vi "GenCM-Read connections.vi"(0 "AO Map":T1, 1 "Path":path, 5 "AI Map":T1, 7 "Digital I-O ref":refnum<vi>, 9 "slot ctl refs":refnum<vi>[](array[refnum]), 11 "error in (no error)":errorcluster, 12 "Analog":cluster{"Inputs":string[], "Outputs":string[]}, 13 "Digital":cluster{"Inputs":string[], "Outputs":string[]}) -> (4 "Hide unused?":bool, 10 "slot ctl refs out":refnum<vi>[](array[refnum]), 15 "error out":errorcluster)   [LabVIEW 2015]
uses:
  Type Defs/General PXISlot XControl/PXISlotGP.xctl
  Type Defs/Digital I-O XControl/Digital I-O.xctl
  PXI DAQ VIs/Utility VIs/Array Dimensions (2D).vi
  <vilib>/Utility/config.llb/Read Key (I32).vi
  <vilib>/Utility/config.llb/Read Key (Boolean).vi
  <vilib>/Utility/config.llb/NI_LVConfig.lvlib
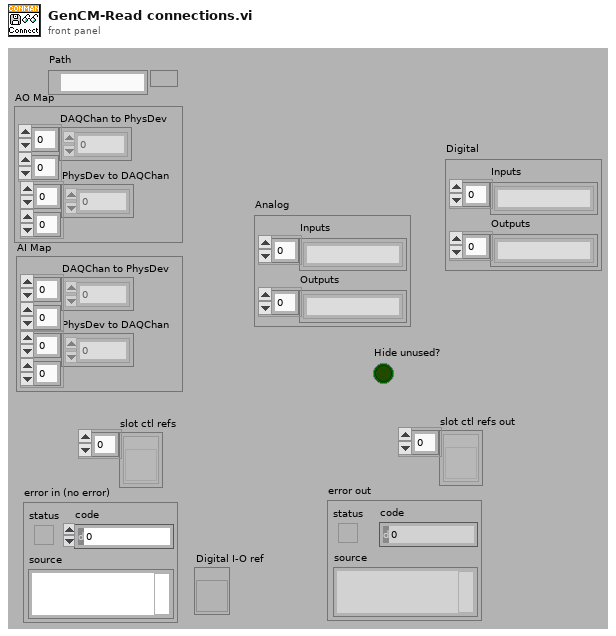
[diagram p1: front panel]
types:
  T1 = cluster{"DAQChan to PhysDev":i32[][], "PhysDev to DAQChan":i32[][]}
  T2 = typedef "NI_LVConfig.lvlib/Config Data RefNum.ctl" = refnum<k1>
  T3 = cluster{"DAQChan to PhysDev":i32[][], "PhysDev to DAQChan":i32[][]}[]
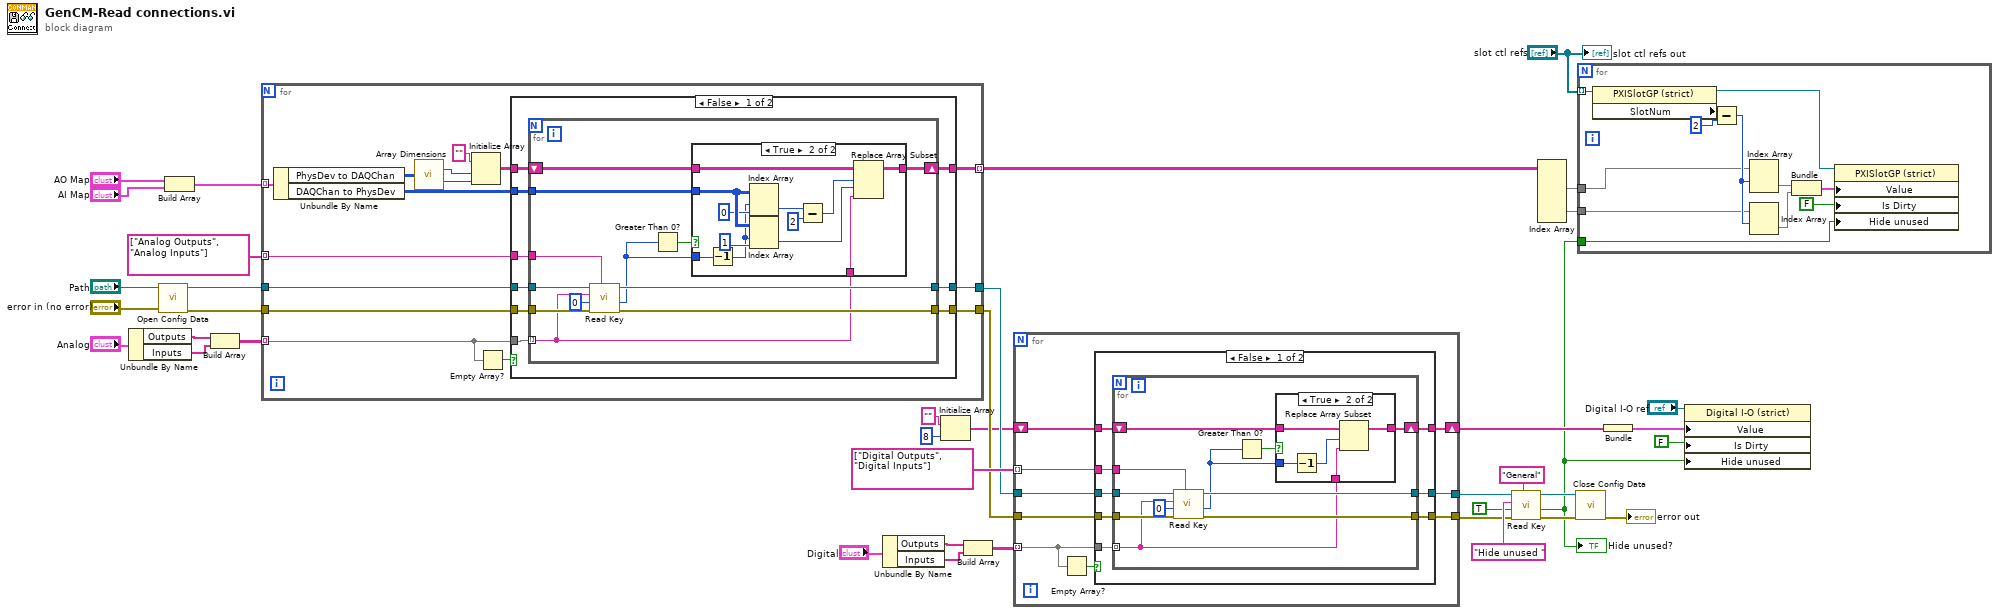
[diagram p0: block diagram]
diagram:
  n1 = Unbundle By Name("Analog") -> ("Outputs"=w25:string[], "Inputs"=w24:string[])
  n2 = call <vilib>:"Open Config Data.vi"("error in (no error)"="error in (no error)", "configuration file path"="Path") -> ("error out"=w31:errorcluster, "refnum"=w38:T2)  [unwired: 7 in, 1 out]
  n3 = Build Array("AO Map", "AI Map") -> (w23:T3)
  n4 = Build Array(w25, w24) -> (w22:string[][])
  n5 = for {
    tunnel: w38 -> [w54]
    tunnel: [w47] -> w20 mode=indexing
    tunnel: [w46] -> w16
    tunnel: w31 -> [w45]
    tunnel: [w44] -> w15
    tunnel: w23 -> [w42] mode=indexing
    tunnel: w22 -> [w41] mode=indexing
    tunnel: string[] ["Analog Outputs", "Analog Inputs"] -> [w40] mode=indexing
    n6 = Unbundle By Name(w42) -> ("PhysDev to DAQChan"=w52:i32[][], "DAQChan to PhysDev"=w53:i32[][])
    n7 = call-poly "Array Dimensions.vi"("2D Array"=w52) -> ("# rows"=w51:i32, "# columns"=w50:i32)  [unwired: 13 in]
    n8 = Initialize Array("" ("element"), w51, w50) -> (w48:string[][])
    n9 = Empty Array?(array=w41) -> (empty?=w43:bool)
    n10 = case shown="False" w43 {
      tunnel: w54 -> [w63 w90]
      tunnel: w53 -> [w62 _]
      tunnel: w48 -> [w61 w91]
      tunnel: [w60 w91] -> w47
      tunnel: [w59 w90] -> w46
      tunnel: w41 -> [w58 _]
      tunnel: w45 -> [w57 w89]
      tunnel: [w56 w89] -> w44
      tunnel: w40 -> [w55 _]
      frame False {
        n11 = for {
          tunnel: w58 -> [w65] mode=indexing
          tunnel: w63 -> [w74]
          tunnel: w62 -> [w72]
          shift-right: [w70] -> w60
          shift-left: w61 -> [w71]
          tunnel: [w69] -> w59
          tunnel: w57 -> [w75]
          tunnel: [w68] -> w56
          tunnel: w55 -> [w64]
          n12 = call-poly <vilib>:"Read Key.vi"("section"=w64, "error in (no error)"=w75, "default value"=0, "key"=w65, "refnum"=w74) -> ("error out"=w68:errorcluster, "value"=w66:i32, "refnum out"=w69:T2)  [unwired: 3 in, 1 out]
          n13 = Greater Than 0?(x=w66) -> (x > 0?=w67:bool)
          n14 = case shown="True" w67 {
            tunnel: w72 -> [_ w88]
            tunnel: w71 -> [w76 w87]
            tunnel: [w76 w86] -> w70
            tunnel: w66 -> [_ w79]
            tunnel: w65 -> [_ w77]
            frame False {
            }
            frame True {
              n15 = Decrement(x=w79) -> (x-1=w78:i32)
              n16 = Index Array(array=w88, index (row)=w78, index (col)=0 ("length")) -> (element=w81:i32)
              n17 = Index Array(array=w88, index (row)=w78, index (col)=1 ("length")) -> (element=w83:i32)
              n18 = Subtract(x=w81, y=2) -> (x-y=w82:i32)
              n19 = Replace Array Subset(array=w87, new element=w77, index (row)=w82, index (col)=w83) -> (w86:string[][])
            }
          }
        }
      }
      frame True {
      }
    }
  }
  n20 = Unbundle By Name("Digital") -> ("Outputs"=w14:string[], "Inputs"=w13:string[])
  n21 = Initialize Array("" ("element"), 8 ("dimension size")) -> (w7:string[])
  n22 = Build Array(w14, w13) -> (w11:string[][])
  n23 = for {
    tunnel: w16 -> [w100]
    tunnel: [w98] -> w1
    tunnel: w15 -> [w97]
    tunnel: [w96] -> w2
    tunnel: w11 -> [w94] mode=indexing
    tunnel: string[] ["Digital Outputs", "Digital Inputs"] -> [w93] mode=indexing
    shift-right: [w99] -> w6
    shift-left: w7 -> [w92]
    n24 = Empty Array?(array=w94) -> (empty?=w95:bool)
    n25 = case shown="False" w95 {
      tunnel: w100 -> [w108 w127]
      tunnel: w92 -> [w107 w128]
      tunnel: [w106 w128] -> w99
      tunnel: [w105 w127] -> w98
      tunnel: w94 -> [w104 _]
      tunnel: w97 -> [w103 w126]
      tunnel: [w102 w126] -> w96
      tunnel: w93 -> [w101 _]
      frame False {
        n26 = for {
          tunnel: w104 -> [w110] mode=indexing
          tunnel: w108 -> [w118]
          shift-right: [w115] -> w106
          shift-left: w107 -> [w116]
          tunnel: [w114] -> w105
          tunnel: w103 -> [w119]
          tunnel: [w113] -> w102
          tunnel: w101 -> [w109]
          n27 = call-poly <vilib>:"Read Key.vi"("section"=w109, "error in (no error)"=w119, "default value"=0, "key"=w110, "refnum"=w118) -> ("error out"=w113:errorcluster, "value"=w111:i32, "refnum out"=w114:T2)  [unwired: 3 in, 1 out]
          n28 = Greater Than 0?(x=w111) -> (x > 0?=w112:bool)
          n29 = case shown="True" w112 {
            tunnel: w116 -> [w120 w125]
            tunnel: [w120 w124] -> w115
            tunnel: w111 -> [_ w123]
            tunnel: w110 -> [_ w122]
            frame False {
            }
            frame True {
              n30 = Decrement(x=w123) -> (x-1=w121:i32)
              n31 = Replace Array Subset(array=w125, new element=w122, index=w121) -> (w124:string[])
            }
          }
        }
      }
      frame True {
      }
    }
  }
  n32 = call-poly <vilib>:"Read Key.vi"("section"="General", "error in (no error)"=w2, "default value"=TRUE, "key"="Hide unused ", "refnum"=w1) -> ("error out"=w36:errorcluster, "value"=w3:bool, "refnum out"=w35:T2)  [unwired: 3 in, 1 out]
  "Hide unused?" <- w3
  n33 = Index Array(array=w20) -> (element #1=w19:string[][], element #2=w18:string[][])  [unwired: 6 in]
  n34 = call <vilib>:"Close Config Data.vi"("error in (no error)"=w36, "refnum"=w35) -> ("error out"=→"error out":errorcluster)  [unwired: 8 in, 1 out]
  n35 = for {
    tunnel: "slot ctl refs" -> [w140] mode=indexing
    tunnel: w19 -> [w132]
    tunnel: w18 -> [w131]
    tunnel: w3 -> [w129]
    n36 = property class="PXISlotGP (strict)"(reference=w140) -> (reference out=w139:refnum<vi>, "SlotNum"=w138:i32)  [unwired: 1 in, 1 out]
    n37 = Subtract(x=w138, y=2) -> (x-y=w135:i32)
    n38 = Index Array(array=w132, index (row)=w135) -> (element=w134:string[])  [unwired: 1 in]
    n39 = Index Array(array=w131, index (row)=w135) -> (element=w136:string[])  [unwired: 1 in]
    n40 = Bundle(w134, w136) -> (w130:cluster{string[], string[]})  [unwired: 1 in]
    n41 = property class="PXISlotGP (strict)"(reference=w139, "Value"=w130, "Is Dirty"=FALSE, "Hide unused"=w129) -> ()  [unwired: 1 in, 2 out]
  }
  n42 = Bundle(w6) -> (w5:cluster{string[]})  [unwired: 1 in]
  n43 = property class="Digital I-O (strict)"(reference="Digital I-O ref", "Value"=w5, "Is Dirty"=FALSE, "Hide unused"=w3) -> ()  [unwired: 1 in, 2 out]
  "slot ctl refs out" <- "slot ctl refs"
